vi "Parcial1ElminMejia.vi"() -> ()   [LabVIEW 2011]
panel:
  out "promedio":dbl
  out "#mayor de gals. generados":dbl
  out "701-1000":bool
  out "501-700":bool
  out "351-500":bool
  out "350 bajo":bool
  in  "Knob":i32(knob) scale=1.0..50.0
  out "tanque":i32(slide) scale=0.0..1000.0
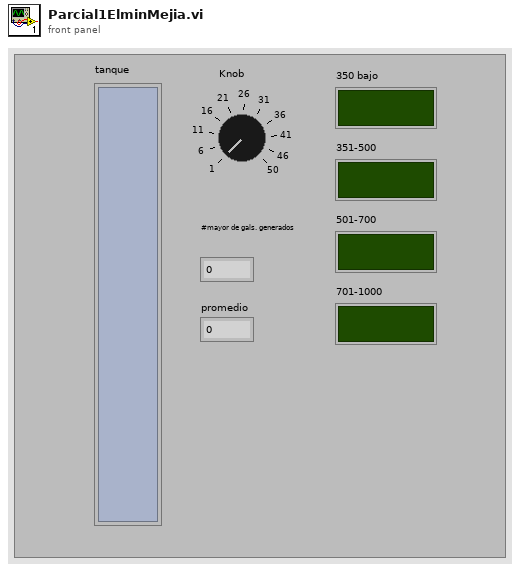
[diagram p1: front panel]
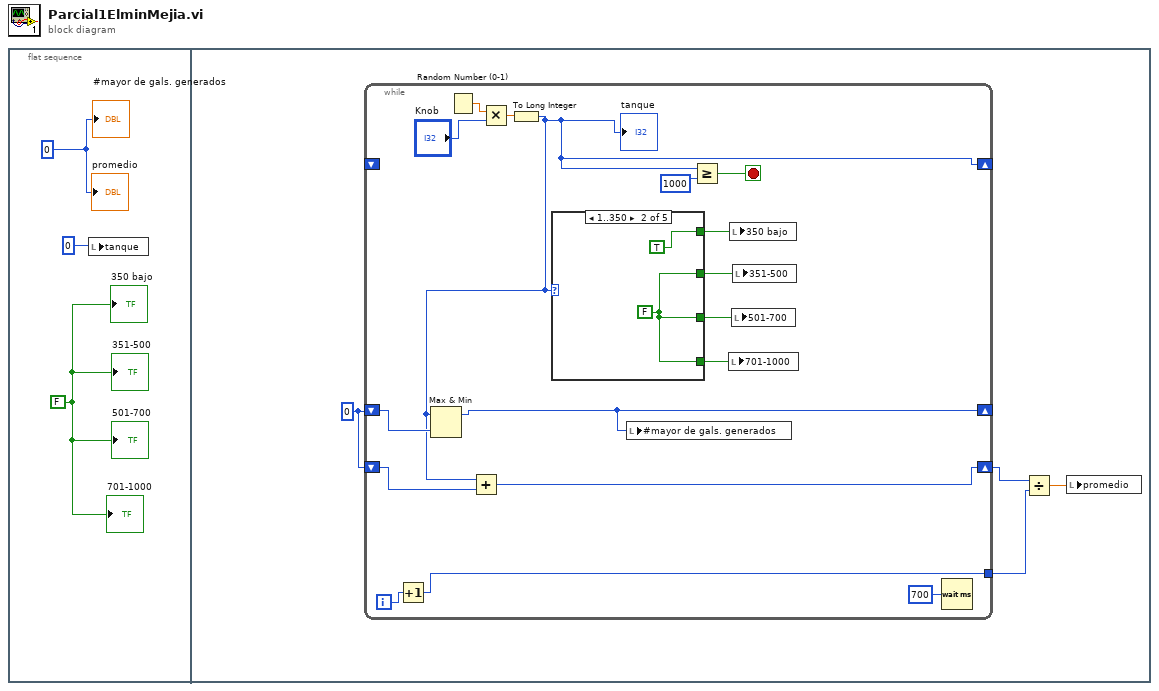
[diagram p0: block diagram]
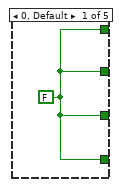
[diagram p2: hidden frame]
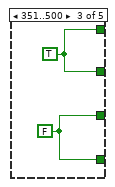
[diagram p3: hidden frame]
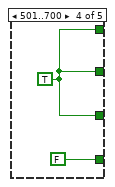
[diagram p4: hidden frame]
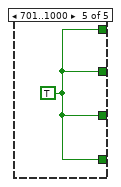
[diagram p5: hidden frame]
diagram:
  n1 = flat-sequence {
    frame #0 {
      w1 = 0
      w3 = FALSE
      n2 = local write "tanque"(0) -> ()
      "350 bajo" <- w3
      "351-500" <- w3
      "501-700" <- w3
      "701-1000" <- w3
      "#mayor de gals. generados" <- w1
      "promedio" <- w1
    }
    frame #1 {
      w7 = 0
      n3 = while {
        shift-right: [w16] -> _
        shift-left: w7 -> [w17]
        shift-right: [w13] -> w4
        shift-left: w7 -> [w14]
        tunnel: [w12] -> w5
        shift-right: [w8] -> _
        shift-left: _ -> [_]
        i -> [w15]
        stop <- w18 stop-if-true
        n4 = Increment(x=w15) -> (x+1=w12:i32)
        n5 = Random Number (0-1)() -> (number: 0 to 1=w11:dbl)
        n6 = Multiply(x=w11, y="Knob") -> (x*y=w10:dbl)
        n7 = To Long Integer(number=w10) -> (32bit integer=w8:i32)
        "tanque" <- w8
        n8 = Max & Min(x=w8, y=w17) -> (max(x,y)=w16:i32)  [unwired: 1 out]
        n9 = Add(x=w8, y=w14) -> (x+y=w13:i32)
        n10 = case shown="1..350" w8 {
          tunnel: [w25 w26 w28 w31 w32] -> w24
          tunnel: [w25 TRUE w29 w31 w32] -> w23
          tunnel: [w25 w26 w29 w31 w32] -> w22
          tunnel: [w25 w26 w28 FALSE w32] -> w21
          frame 0, Default {
            w25 = FALSE
          }
          frame 1..350 {
            w26 = FALSE
          }
          frame 351..500 {
            w28 = FALSE
            w29 = TRUE
          }
          frame 501..700 {
            w31 = TRUE
          }
          frame 701..1000 {
            w32 = TRUE
          }
        }
        n11 = local write "#mayor de gals. generados"(w16) -> ()
        n12 = Greater Or Equal?(x=w8, y=1000) -> (x >= y?=w18:bool)
        n13 = local write "701-1000"(w21) -> ()
        n14 = local write "350 bajo"(w23) -> ()
        n15 = local write "501-700"(w24) -> ()
        n16 = local write "351-500"(w22) -> ()
        n17 = Wait (ms)(milliseconds to wait=u32 700) -> ()  [unwired: 1 out]
      }
      n18 = Divide(x=w4, y=w5) -> (x/y=w6:dbl)
      n19 = local write "promedio"(w6) -> ()
    }
  }
